vi "Get Stop Notifier.vi"(8 "error in (no error)":errorcluster, 11 "Transport in":refnum<class "Transport.lvclass">) -> (0 "error out":errorcluster, 2 "Stop?":bool, 3 "Transport out":refnum<class "Transport.lvclass">)   [LabVIEW 2019, in "Transport.lvclass"]
uses:
  Transport.lvclass
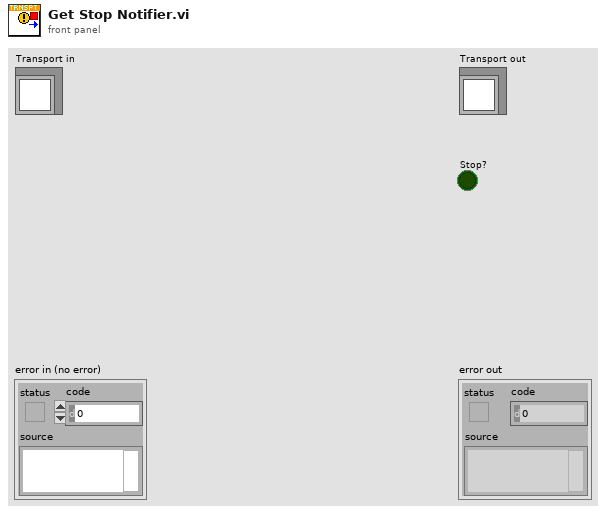
[diagram p1: front panel]
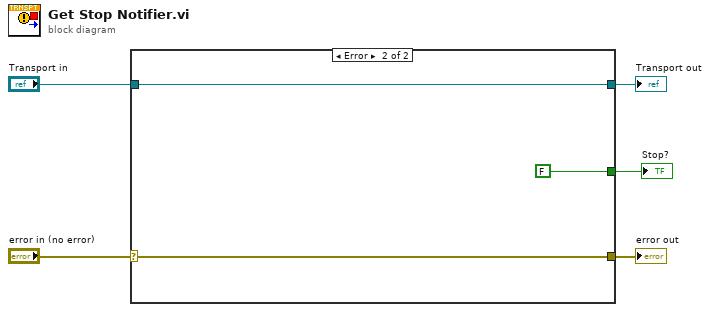
[diagram p0: block diagram]
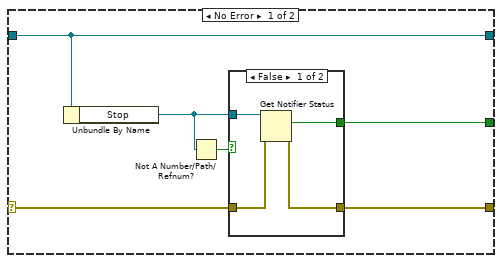
[diagram p2: hidden frame]
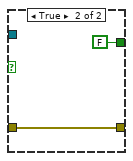
[diagram p3: hidden frame]
diagram:
  n1 = case shown="Error" "error in (no error)" {
    selector: "error in (no error)" -> [w11 w19]
    tunnel: [w10 w19] -> w4
    tunnel: [w8 w20] -> w2
    tunnel: "Transport in" -> [w8 w20]
    tunnel: [w9 FALSE] -> w1
    frame No Error {
      n2 = Unbundle By Name(w8) -> ("Stop"=w7:refnum<notifier>)
      n3 = Not A Number/Path/Refnum?(number/path/refnum=w7) -> (NaN/Path/Refnum?=w6:bool)
      n4 = case shown="False" w6 {
        tunnel: w11 -> [w15 w16]
        tunnel: [w14 w16] -> w10
        tunnel: [w13 FALSE] -> w9
        tunnel: w7 -> [w12 _]
        frame False {
          n5 = Get Notifier Status(notifier=w12, error in (no error)=w15) -> (current notification=w13:bool, error out=w14:errorcluster)  [unwired: 3 out]
        }
        frame True {
        }
      }
    }
    frame Error {
    }
  }
  "error out" <- w4
  "Transport out" <- w2
  "Stop?" <- w1
